vi "DFD Analyze Filter Bank Distortion.vi"(6 "fs in [Hz]":dbl=-1.0, 7 "# freq bins":i32=-1, 8 "error in (no error)":errorcluster, 9 "dB on? (T)":bool=TRUE, 10 "phase view":T9, 11 "filter bank in":T1={"mFBank_AnalysisFilters"=[], "mFBank_SynthesisFilters"=[], "mFBank_#Bands"=2, "mFBank_ProcMethod"=enum."General", "mFBank_Coeffs"=[], "mFBank_Gain"=1.0, "mFBank_Delay"=0, "mFBank_Type"=0} {"mFBank_SynthesisFilters"."mMRate_SumWl" min=1 max=32 step=1; "mFBank_SynthesisFilters"."mMRate_InputIwl" min=1 max=32 step=1; "mFBank_SynthesisFilters"."mMRate_GainWl" min=1 max=32 step=1; "mFBank_SynthesisFilters"."mMRate_OutputWl" min=1 max=32 step=1; "mFBank_SynthesisFilters"."mMRate_InputWl" min=1 max=32 step=1; "mFBank_SynthesisFilters"."mMRate_CoefWl" min=1 max=32 step=1; "mFBank_SynthesisFilters"."mMRate_Mode" items=["Default"=-1, "No Rate Change"=0, "Interpolation"=1, "Decimation"=2, "Interpolated"=3, "Rational"=4]; "mFBank_AnalysisFilters"."mMRate_SumWl" min=1 max=32 step=1; "mFBank_AnalysisFilters"."mMRate_InputIwl" min=1 max=32 step=1; "mFBank_AnalysisFilters"."mMRate_GainWl" min=1 max=32 step=1; "mFBank_AnalysisFilters"."mMRate_OutputWl" min=1 max=32 step=1; "mFBank_AnalysisFilters"."mMRate_InputWl" min=1 max=32 step=1; "mFBank_AnalysisFilters"."mMRate_CoefWl" min=1 max=32 step=1; "mFBank_AnalysisFilters"."mMRate_Mode" items=["Default"=-1, "No Rate Change"=0, "Interpolation"=1, "Decimation"=2, "Interpolated"=3, "Rational"=4]; "mFBank_Type" items=["Uniform", "Non-Uniform"]}) -> (0 "error out":errorcluster, 1 "magnitude distortion":cluster{dbl[], "values":dbl[]}(graph), 2 "aliasing":cluster{dbl[], "values":dbl[]}(graph), 3 "filter bank out":T1={"mFBank_AnalysisFilters"=[], "mFBank_SynthesisFilters"=[], "mFBank_#Bands"=2, "mFBank_ProcMethod"=enum."General", "mFBank_Coeffs"=[], "mFBank_Gain"=1.0, "mFBank_Delay"=0, "mFBank_Type"=0} {"mFBank_SynthesisFilters"."mMRate_SumWl" min=1 max=32 step=1; "mFBank_SynthesisFilters"."mMRate_InputIwl" min=1 max=32 step=1; "mFBank_SynthesisFilters"."mMRate_GainWl" min=1 max=32 step=1; "mFBank_SynthesisFilters"."mMRate_OutputWl" min=1 max=32 step=1; "mFBank_SynthesisFilters"."mMRate_InputWl" min=1 max=32 step=1; "mFBank_SynthesisFilters"."mMRate_CoefWl" min=1 max=32 step=1; "mFBank_SynthesisFilters"."mMRate_Mode" items=["Default"=-1, "No Rate Change"=0, "Interpolation"=1, "Decimation"=2, "Interpolated"=3, "Rational"=4]; "mFBank_AnalysisFilters"."mMRate_SumWl" min=1 max=32 step=1; "mFBank_AnalysisFilters"."mMRate_InputIwl" min=1 max=32 step=1; "mFBank_AnalysisFilters"."mMRate_GainWl" min=1 max=32 step=1; "mFBank_AnalysisFilters"."mMRate_OutputWl" min=1 max=32 step=1; "mFBank_AnalysisFilters"."mMRate_InputWl" min=1 max=32 step=1; "mFBank_AnalysisFilters"."mMRate_CoefWl" min=1 max=32 step=1; "mFBank_AnalysisFilters"."mMRate_Mode" items=["Default"=-1, "No Rate Change"=0, "Interpolation"=1, "Decimation"=2, "Interpolated"=3, "Rational"=4]; "mFBank_Type" items=["Uniform", "Non-Uniform"]}, 4 "phase distortion":cluster{dbl[], "values":dbl[]}(graph))   [LabVIEW 2017, in "NI_DigFilter_FilterBank.lvlib"]
doc: "Evaluates whether a filter bank is a perfect reconstruction filter bank or near-perfect reconstruction filter bank. This VI analyzes the three fundamental distortions in filter banks: aliasing, magnitude distortion, and phase distortion. You also can use this VI to evaluate filter banks that the Filter Bank Design VIs and the DFD Build Filter Bank from Prototype Filter VI create."
uses:
  <vilib>/addons/Digital Filter Design/NI_DigFilter_FilterBank.lvlib
  <vilib>/addons/Digital Filter Design/_Objects.llb/DFD Phase Setting.ctl
  <vilib>/addons/Digital Filter Design/FilterBank.llb/Object/DFD Filter Bank Obj.ctl
  <vilib>/addons/Digital Filter Design/_Objects.llb/DFD Multirate Filter Obj.ctl
  <vilib>/addons/Digital Filter Design/_Objects.llb/DFD Multirate Mode.ctl
  <vilib>/addons/Digital Filter Design/_Objects.llb/DFD Coef Norm Type.ctl
  <vilib>/addons/Digital Filter Design/_Objects.llb/DFD Round-off Mode.ctl
  <vilib>/addons/Digital Filter Design/_Objects.llb/DFD FXP MRate Multiply Mode.ctl
  <vilib>/addons/Digital Filter Design/FilterBank.llb/Object/DFD Filter Bank Processing Method.ctl
  <vilib>/addons/Digital Filter Design/FilterBank.llb/Object/DFD Filter Bank Type.ctl
  <vilib>/addons/Digital Filter Design/NI_DigFilterLicensed.lvlib
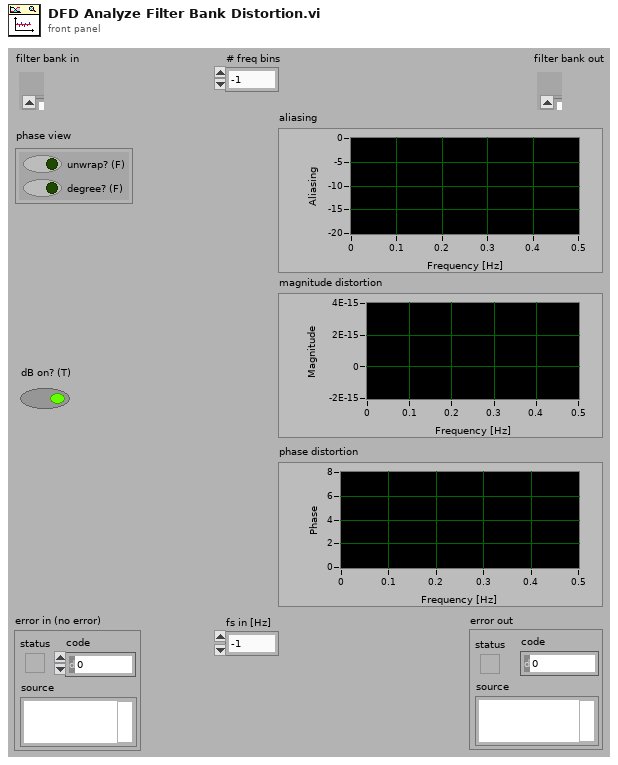
[diagram p1: front panel]
types:
  T1 = typedef "NI_DigFilter_FilterBank.lvlib/DFD Filter Bank Obj.ctl" = cluster{"mFBank_AnalysisFilters":T2[], "mFBank_SynthesisFilters":T2[], "mFBank_#Bands":i32, "mFBank_ProcMethod":T7, "mFBank_Coeffs":dbl[], "mFBank_Gain":dbl, "mFBank_Delay":i32, "mFBank_Type":T8}
  T2 = typedef "NI_DigFilterLicensed.lvlib/DFD Multirate Filter Obj.ctl" = cluster{"mMRate_Structure":enum16{"CIC", "FIR", "IIR", "Lattice"}, "mMRate_Mode":T3, "mMRate_Factor":i32, "mMRate_FIRParams":cluster{"mMRate_FIR_H":dbl[], "mMRate_FIR_IsNyquist?":bool, "mMRate_FIR_IsSymmetric?":bool}, "mMRate_CICParams":cluster{"mMRate_CIC_#Stage":i32, "mMRate_CIC_Lag":i32, "mMRate_CIC_Type":enum16{"Lowpass", "Highpass"}}, "mMRate_Order":i32, "mMRate_Version":string, "mMRate_Comments":string, "mMRate_RationalFactor":cluster{"mMRate_L":i32, "mMRate_M":i32}, "mMRate_Fs":dbl, "mMRate_Quantized?":bool, "mMRate_QFilterGain":dbl, "mMRate_CoefWl":i16, "mMRate_Scaling":cluster{"mMRate_ScaleByPowerOf2?":bool, "mMRate_ScaleType":T4}, "mMRate_InputWl":i16, "mMRate_OutputWl":i16, "mMRate_OutputMode":T5, "mMRate_MultMode":T6, "mMRate_BitPruning":bool, "mMRate_GainWl":i16, "mMRate_OutputFwl":i16, "mMRate_SumIwl":i16, "mMRate_InputIwl ":i16, "mMRate_SumWl":i16, "mMRate_CoefIwl":i16}
  T3 = typedef "NI_DigFilterLicensed.lvlib/DFD Multirate Mode.ctl" = i16
  T4 = typedef "NI_DigFilterLicensed.lvlib/DFD Coef Norm Type.ctl" = enum16{"No Norm", "Time Domain 1-Norm", "Time Domain 2-Norm", "Time Domain Inf-Norm"}
  T5 = typedef "NI_DigFilterLicensed.lvlib/DFD Round-off Mode.ctl" = enum16{"Nearest", "Truncation"}
  T6 = typedef "NI_DigFilterLicensed.lvlib/DFD FXP MRate Multiply Mode.ctl" = enum16{"Truncated", "Full"}
  T7 = typedef "NI_DigFilter_FilterBank.lvlib/DFD Filter Bank Processing Method.ctl" = enum16{"General", "2-Band QMF Lattice", "Cosine-Modulated"}
  T8 = typedef "NI_DigFilter_FilterBank.lvlib/DFD Filter Bank Type.ctl" = u16
  T9 = typedef "NI_DigFilterLicensed.lvlib/DFD Phase Setting.ctl" = cluster{"unwrap? (F)":bool, "degree? (F)":bool}
  T10 = typedef "NI_DigFilter_FilterBank.lvlib/DFD Bank Obj.ctl" = cluster{"mBank_Filters":T2[], " mBank_#Bands":i32, "mBank_ProcMethod":T7, "mBank_Coeffs":dbl[], "mBank_Gain":dbl, "mBank_Type":T8}
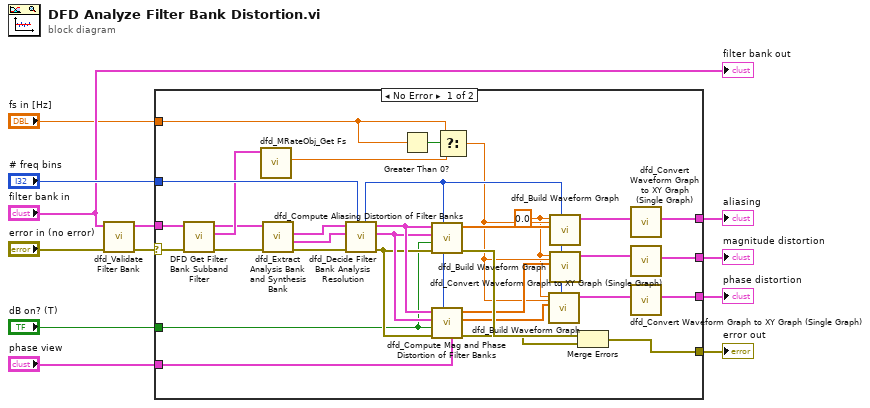
[diagram p0: block diagram]
diagram:
  n1 = call <vilib>:"dfd_Validate Filter Bank.vi"("error in (no error)"="error in (no error)", "filter banks in"="filter bank in") -> ("error out"=w5:errorcluster, "filter bank out"=w4:T1)  [unwired: 7 in, 1 out]
  n2 = case shown="No Error" w5 {
    selector: w5 -> [w28 w45]
    tunnel: "# freq bins" -> [w43 _]
    tunnel: [w32 _] -> w7
    tunnel: [w36 w45] -> w11
    tunnel: "dB on? (T)" -> [w35 _]
    tunnel: "phase view" -> [w44 _]
    tunnel: [w33 _] -> w8
    tunnel: w4 -> [w29 _]
    tunnel: [w34 _] -> w2
    tunnel: "fs in [Hz]" -> [w22 _]
    frame No Error {
      w13 = 0.0 ("f0")
      n3 = call <vilib>:"DFD Get Filter Bank Subband Filter.vi"("error in (no error)"=w28, "filter bank in"=w29) -> ("error out"=w25:errorcluster, "subband filter"=w27:T2, "filter bank out"=w26:T1)  [unwired: 7 in]
      n4 = call <vilib>:"dfd_MRateObj_Get Fs.vi"("multirate filter in"=w27) -> ("fs"=w23:dbl)  [unwired: 10 out]
      n5 = call <vilib>:"dfd_Extract Analysis Bank and Synthesis Bank.vi"("error in (no error)"=w25, "filter banks in"=w26) -> ("error out"=w30:errorcluster, "synthesis bank"=w42:T10, "analysis bank"=w31:T10)  [unwired: 6 in, 1 out]
      n6 = call <vilib>:"dfd_Decide Filter Bank Analysis Resolution.vi"("# freq bins in"=w43, "error in (no error)"=w30, "synthesis bank in"=w42, "analysis bank in"=w31) -> ("error out"=w39:errorcluster, "synthesis bank out"=w40:T10, "analysis bank out"=w41:T10, "# freq bins out"=w18:i32)  [unwired: 4 in]
      n7 = Greater Than 0?(x=w22) -> (x > 0?=w24:bool)
      n8 = call <vilib>:"dfd_Compute Aliasing Distortion of Filter Banks.vi"("# freq bins"=w18, "error in (no error)"=w39, "dB on? (T)"=w35, "synthesis bank"=w40, "analysis bank"=w41) -> ("error out"=w38:errorcluster, "aliasing distortion"=w21:dbl[])  [unwired: 5 in]
      n9 = call <vilib>:"dfd_Compute Mag and Phase Distortion of Filter Banks.vi"("phase view"=w44, "# freq bins"=w18, "error in (no error)"=w39, "dB on? (T)"=w35, "synthesis bank"=w40, "analysis bank"=w41) -> ("error out"=w37:errorcluster, "phase"=w16:dbl[], "amplitude"=w19:dbl[])  [unwired: 3 in]
      n10 = Select(t=w22, s=w24, f=w23) -> (s? t:f=w17:dbl)
      n11 = call <vilib>:"dfd_Build Waveform Graph.vi"("fs"=w17, "# freq bins out"=w18, "values"=w16, "f0"=w13) -> ("waveform"=w15:cluster{"f0":dbl, "df":dbl, "values":dbl[]})  [unwired: 7 in]
      n12 = call <vilib>:"dfd_Build Waveform Graph.vi"("fs"=w17, "# freq bins out"=w18, "values"=w21, "f0"=w13) -> ("waveform"=w20:cluster{"f0":dbl, "df":dbl, "values":dbl[]})  [unwired: 7 in]
      n13 = call <vilib>:"dfd_Build Waveform Graph.vi"("fs"=w17, "# freq bins out"=w18, "values"=w19, "f0"=w13) -> ("waveform"=w14:cluster{"f0":dbl, "df":dbl, "values":dbl[]})  [unwired: 7 in]
      n14 = Merge Errors(w38, w37) -> (w36:errorcluster)
      n15 = call <vilib>:"dfd_Convert Waveform Graph to XY Graph (Single Graph).vi"("waveform"=w20) -> ("XY graph"=w34:cluster{dbl[], "values":dbl[]})  [unwired: 10 in]
      n16 = call <vilib>:"dfd_Convert Waveform Graph to XY Graph (Single Graph).vi"("waveform"=w14) -> ("XY graph"=w32:cluster{dbl[], "values":dbl[]})  [unwired: 10 in]
      n17 = call <vilib>:"dfd_Convert Waveform Graph to XY Graph (Single Graph).vi"("waveform"=w15) -> ("XY graph"=w33:cluster{dbl[], "values":dbl[]})  [unwired: 10 in]
    }
    frame Error {
    }
  }
  "error out" <- w11
  "magnitude distortion" <- w7
  "phase distortion" <- w8
  "aliasing" <- w2
  "filter bank out" <- "filter bank in"
